vi "Convert to 3D.vi"(7 "Degrees per pixel (0.1)":dbl=0.1009937888, 9 "Y Resolution (480)":i32=480, 10 "X Resolution (640)":i32=640, 11 "Depth image":i32[][](array[numeric])) -> (1 "z Values":dbl[][](array[numeric]), 2 "y Values":dbl[][](array[numeric]), 3 "x Values":dbl[][](array[numeric]))   [LabVIEW 2010]
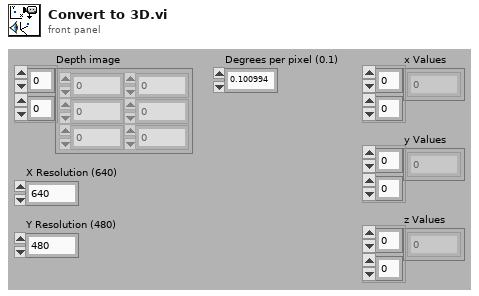
[diagram p1: front panel]
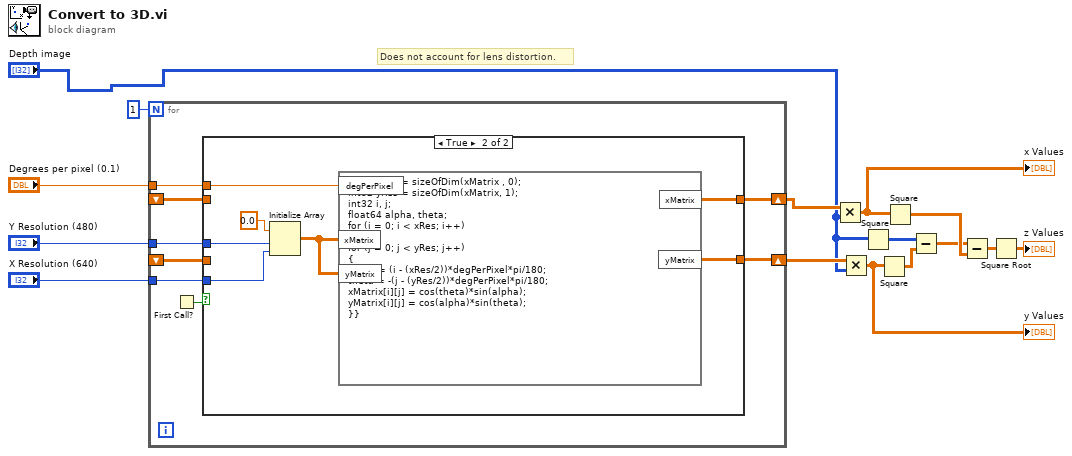
[diagram p0: block diagram]
diagram:
  # "Does not account for lens distortion."
  n1 = for {
    N: 1 -> [_]
    tunnel: "Degrees per pixel (0.1)" -> [w23]
    tunnel: "Y Resolution (480)" -> [w22]
    tunnel: "X Resolution (640)" -> [w21]
    shift-right: [w18] -> w11
    shift-left: _ -> [w16]
    shift-right: [w19] -> w10
    shift-left: _ -> [w17]
    n2 = First Call?() -> (First Call?: T/F=w20:bool)
    n3 = case shown="True" w20 {
      tunnel: w23 -> [_ w32]
      tunnel: w22 -> [_ w31]
      tunnel: w21 -> [_ w30]
      tunnel: [w25 w27] -> w19
      tunnel: [w24 w26] -> w18
      tunnel: w17 -> [w25 _]
      tunnel: w16 -> [w24 _]
      frame False {
      }
      frame True {
        n4 = Initialize Array(0.0, w31, w30) -> (w28:dbl[][])
        n5 = formula code="int32 xRes = sizeOfDim(xMatrix , 0);\nint32 yRes = sizeOfDim(xMatrix, 1);\nint32 i, j; \nfloat64 alpha, theta;\nfor (i = 0; i < xRes; i++)\n{\nfor (j = 0; j < yRes; j++)\n{\nalpha = (i - (xRes/2))*degPerPixel*pi/180;\ntheta = -(j - (yRes/2))*degPerPixel*pi/180;\nxMatrix[i][j] = cos(theta)*sin(alpha);\nyMatrix[i][j] = cos(alpha)*sin(theta);\n}}"("degPerPixel"=w32, "xMatrix"=w28, "yMatrix"=w28) -> ("xMatrix"=w27:dbl[][], "yMatrix"=w26:dbl[][])
      }
    }
  }
  n6 = Multiply(x=w10, y="Depth image") -> (x*y=w7:dbl[][])
  "x Values" <- w7
  n7 = Multiply(x=w11, y="Depth image") -> (x*y=w3:dbl[][])
  "y Values" <- w3
  n8 = Square(x="Depth image") -> (x^2=w8:i32[][])
  n9 = Square(x=w3) -> (x^2=w9:dbl[][])
  n10 = Square(x=w7) -> (x^2=w6:dbl[][])
  n11 = Subtract(x=w8, y=w9) -> (x-y=w5:dbl[][])
  n12 = Subtract(x=w5, y=w6) -> (x-y=w4:dbl[][])
  n13 = Square Root(x=w4) -> (sqrt(x)=→"z Values":dbl[][])
